vi "Magnet Gap Tester (FPGA).vi"() -> ()   [LabVIEW 2019]
uses:
  <vilib>/Platform/TimedLoop/XDataNode/wakeup.ctl
  <vilib>/Platform/TimedLoop/XDataNode/XDNodeRunTimeDep.lvlib
  <vilib>/Platform/TimedLoop/XDataNode/nitl_modes.ctl
  <vilib>/Platform/TimedLoop/XDataNode/timing_clust.ctl
  <vilib>/Platform/TimedLoop/XDataNode/XDataNode.xnode
  <vilib>/eio/EIONode/EIONode.xnode
  <vilib>/rvi/eio/common/nirviEmuTemplateMethod_errors.vi
  <vilib>/rvi/DataTransferAndStorage/Container/XNode/niFpgaContainer.xnode
  <vilib>/rvi/interface/RandomDataEmulation/nirviRandomDataFpgaReadWriteTemplate.vi
  <vilib>/eio/EIOMethodNode/EIOMethodNode.xnode
  Controls/i2c_state.ctl
panel:
  in  "Samples to Avg":i16=10
  out "AI0":fxp<+/-,24,5>
  in  "Execute":bool
  in  "HalfCycle(Ticks)":u32=200
  in  "i2c_State":T1=enum."W_To_Device"
  in  "Address":u8 format="%08x"
  in  "10-bitAddress":u8 format="%08b"
  in  "TransmitDelay(Ticks)":u32=1000
  in  "Use_10-Bit_Address":bool
  in  "StartStopDelay(Ticks)":u32=1200
  in  "PostAddressDelay(Ticks)":u32=1200
  in  "NumBytesToWrite":i32
  in  "NumBytesToRead":i32
  out "error":errorcluster
  out "Status":i16
  in  "CMD/Param":u8 format="%.0x"
  out "Data":u8 format="%.0x"
  in  "MemoryAddress":u32
  in  "GetRead":bool
  in  "UpdateWrite":bool
  out "REV OUT":bool
  out "FWD OUT":bool
  in  "Reverse":bool
  in  "Forward":bool
  in  "Motor Stop Offset":i32=589
  in  "REV Limit":i32=589
  in  "FWD Limit":i32=589
  out "AI0 (avg)":fxp<+/-,24,5> format="%.4g"
  in  "AI Loop (uSec)":u32
  out "AI Loop Actual":u32=20
  in  "Position Reset":bool
  out "Position (Counts)":i32=589
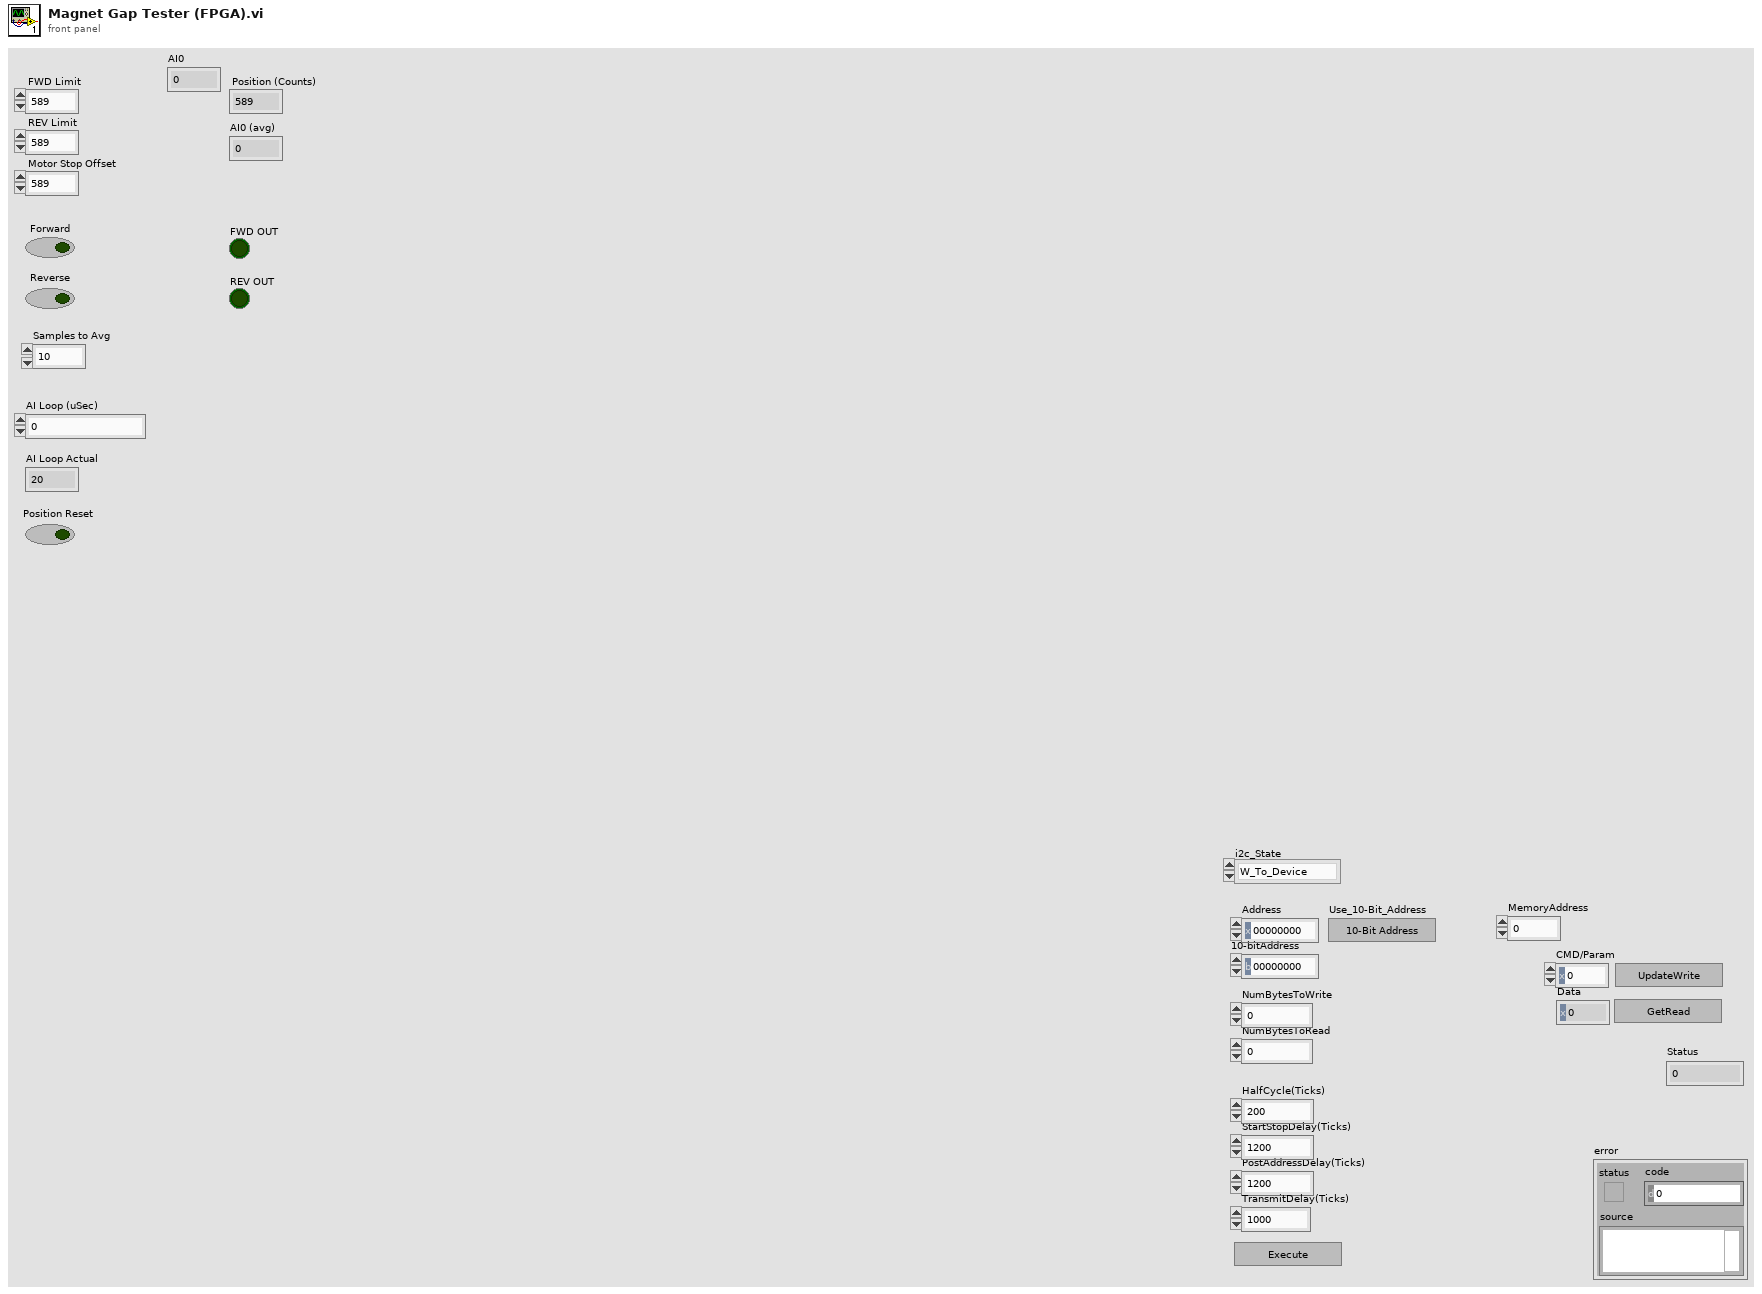
[diagram p1: front panel]
types:
  T1 = typedef "i2c_state.ctl" = enum16{"Monitor", "W_To_Device", "R_From_Device", "W/R_From_Device", "TerminateCore"}
  T2 = typedef "XDNodeRunTimeDep.lvlib/timing_clust.ctl" = cluster{"Expected End [f-1]":u64, "Actual End [f-1]":u64, "Finished Late? [f-1]":bool, "Expected End [i-1]":u64, "Actual End [i-1]":u64, "Finished Late? [i-1]":bool, "Expected Start [i]":u64, "Actual Start [i]":u64, "Expected Start [f]":u64, "Actual Start [f]":u64, "Source Name":string, "Structure Name":string, "Period":i64, "Deadline":i64, "Offset":i64, "Start":i64, "Priority":i32, "Timeout":i32, "Mode":T3, "Wakeup Reason":T4, "Error":errorcluster, "Source Type":string, "Secondary Source Type":string, "Global End Time":u64, "Global Start Time":u64, "Frame Duration":u64, "Iteration Duration":u64, "Assigned CPU":i32, "I/O Scan Engine Mode":u32}
  T3 = typedef "XDNodeRunTimeDep.lvlib/nitl_modes.ctl" = enum32{"No Change", "Process missed periods, maintain original phase", "Discard missed periods, maintain original phase", "Process missed periods, ignore original phase", "Discard missed periods, ignore original phase"}
  T4 = typedef "XDNodeRunTimeDep.lvlib/wakeup.ctl" = enum32{"Normal", "Aborted", "Asynchronous wakeup", "Timing source error", "Timed loop error", "Timeout"}
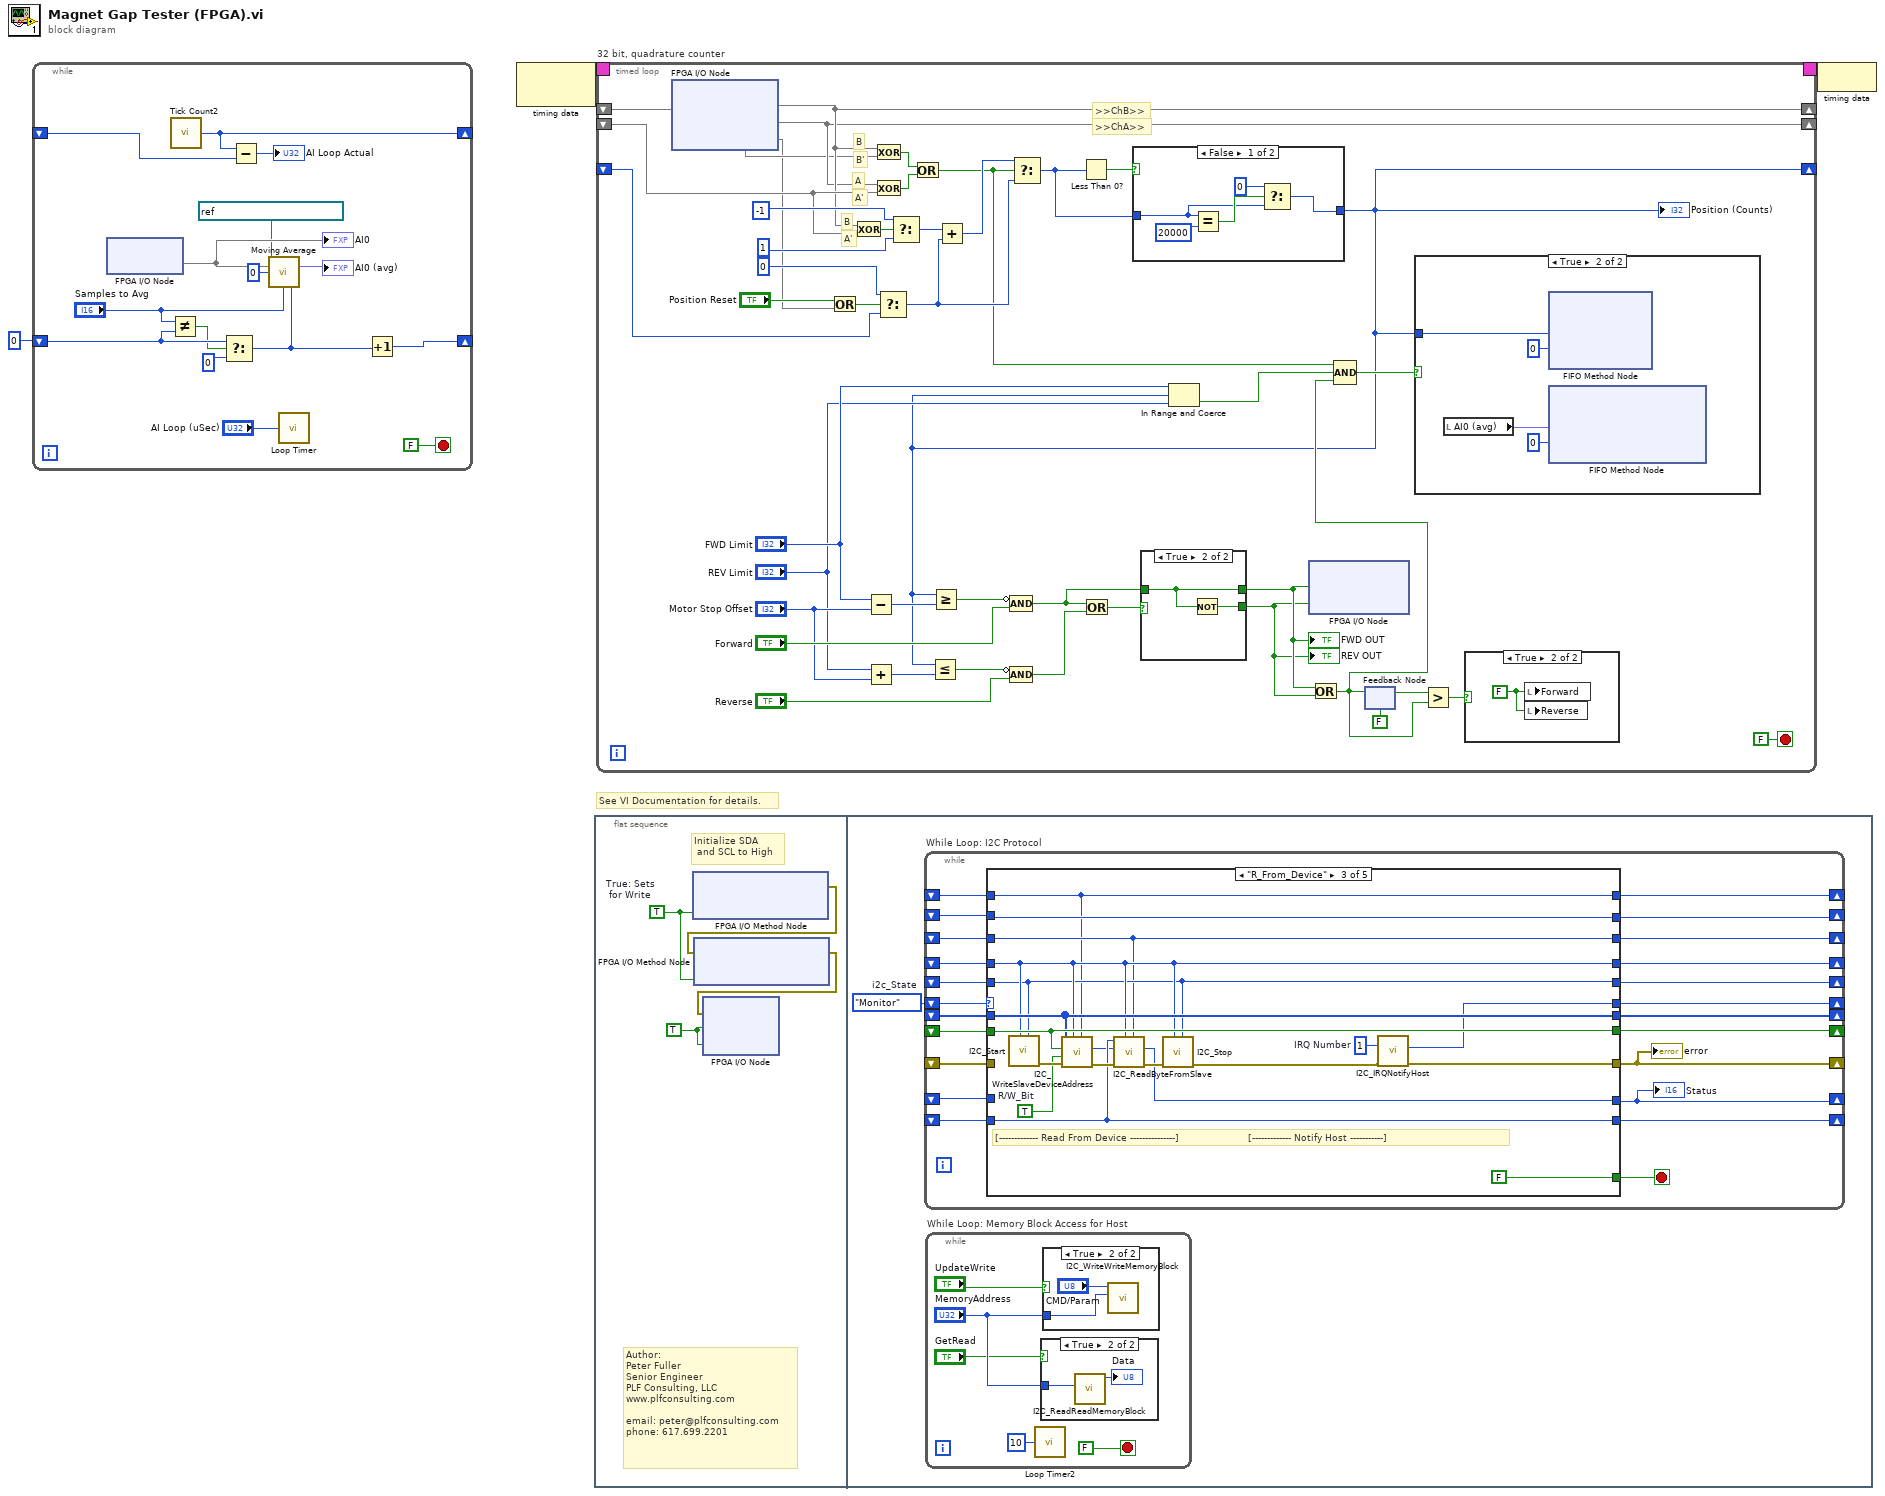
[diagram p0: block diagram]
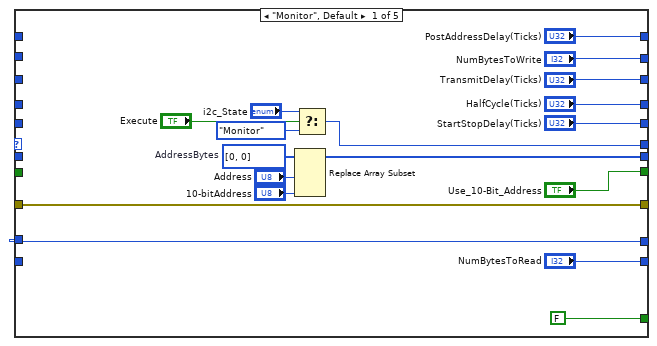
[diagram p4: hidden frame]
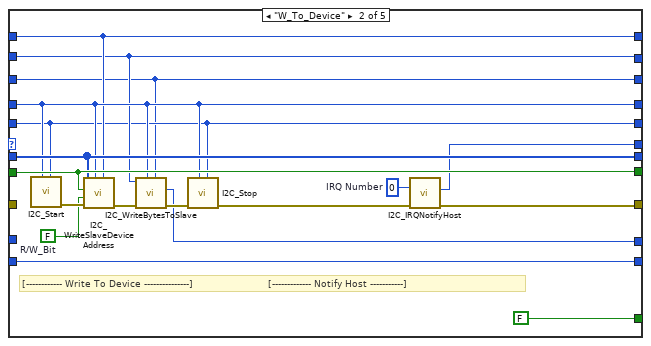
[diagram p5: hidden frame]
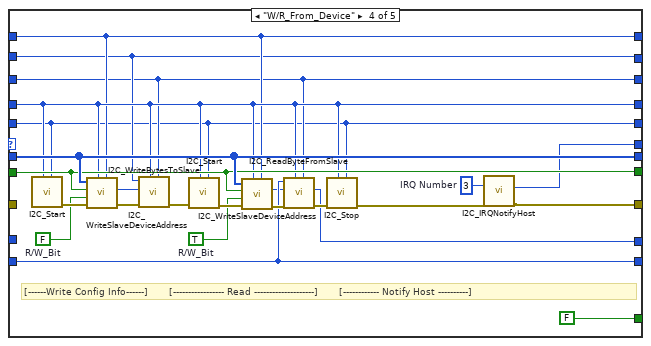
[diagram p6: hidden frame]
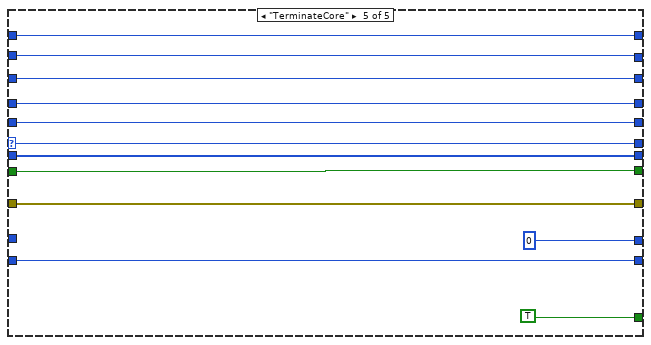
[diagram p7: hidden frame]
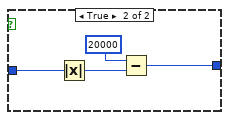
[diagram p11: hidden frame]
diagram:
  # "See VI Documentation for details."
  n1 = while {
    shift-right: [w16] -> _
    shift-left: _ -> [w15]
    shift-right: [w8] -> _
    shift-left: i16 0 ("Moving Point Index") -> [w7]
    stop <- FALSE stop-if-true
    n2 = xnode "FPGA I/O Node"() -> ("AI0"=w13)  [unwired: 1 in, 1 out]
    "AI0" <- w13
    n3 = Not Equal?(x="Samples to Avg", y=w7) -> (x != y?=w5:bool)
    n4 = call "Tick Count2"() -> ("Tick Count(uSec)"=w16:u32)
    n5 = Select(t=w7, s=w5, f=i16 0) -> (s? t:f=w9:i16)
    n6 = Subtract(x=w16, y=w15) -> (x-y=→"AI Loop Actual":u32)
    n7 = call "Moving Average.vi"("Memory In"=refnum<k21> "Running Avg Memory", "N (# of Ave Pts 127 max)"="Samples to Avg", "Moving Point Index"=w9, "Data IN"=w13, "Channel#"=i16 0) -> ("Averaged Data"=→"AI0 (avg)":fxp<+/-,28,17>)  [unwired: 10 in]
    n8 = call "Loop Timer"("Count(uSec)"="AI Loop (uSec)") -> ()  [unwired: 1 out]
    n9 = Increment(x=w9) -> (x+1=w8:i16)
  }
  n10 = node-c288() -> (w3:T2)  [unwired: 1 in]
  n11 = flat-sequence {
    frame #0 {
      w20 = TRUE  # True: Sets   for Write
      w22 = TRUE ("SDA")
      # "Author:\nPeter Fuller\nSenior Engineer\nPLF Consulting, LLC\nwww.plfconsulting.com\n\nemail: peter@plfconsulting.com\nphone: 617.699.2201"
      # "Initialize SDA\n and SCL to High"
      n12 = xnode "FPGA I/O Method Node"("Enable"=w20) -> ("error out"=w21:errorcluster)  [unwired: 2 in, 1 out]
      n13 = xnode "FPGA I/O Method Node"("error in"=w21, "Enable"=w20) -> ("error out"=w19:errorcluster)  [unwired: 1 in, 1 out]
      n14 = xnode "FPGA I/O Node"("error in"=w19, "SDA"=w22, "SCL"=w22) -> ()  [unwired: 2 in, 3 out]
    }
    frame #1 {
      w23 = i2c_state."Monitor"  # i2c_State
      n15 = while "While Loop: I2C Protocol" {
        shift-right: [w50] -> _
        shift-left: w23 -> [w51]
        shift-right: [w54] -> _
        shift-left: _ -> [w55]
        shift-right: [w35] -> _
        shift-left: _ -> [w53]
        shift-right: [w49] -> _
        shift-left: _ -> [w52]
        shift-right: [w48] -> _
        shift-left: _ -> [w47]
        shift-right: [w46] -> _
        shift-left: _ -> [w45]
        shift-right: [w43] -> _
        shift-left: _ -> [w39]
        shift-right: [w42] -> _
        shift-left: _ -> [w38]
        shift-right: [w41] -> _
        shift-left: _ -> [w36]
        shift-right: [w40] -> _
        shift-left: _ -> [w37]
        shift-right: [w34] -> _
        shift-left: _ -> [w33]
        stop <- w44 stop-if-true
        n16 = case shown="\"R_From_Device\"" w51 {
          selector: w51 -> [_ _ _ _ w139]
          tunnel: ["HalfCycle(Ticks)" w88 w105 w126 w141] -> w54
          tunnel: w55 -> [_ w88 w105 w126 w141]
          tunnel: [w69 w83 w92 w111 w139] -> w50
          tunnel: w53 -> [w57 _ _ _ w145]
          tunnel: [w57 w76 w93 w112 w145] -> w35
          tunnel: w52 -> [_ w89 w108 w131 w138]
          tunnel: [w65 w89 w108 w131 w138] -> w49
          tunnel: ["Use_10-Bit_Address" w90 w109 w130 w137] -> w48
          tunnel: w47 -> [_ w90 w109 w130 w137]
          tunnel: ["TransmitDelay(Ticks)" w77 w99 w119 w142] -> w46
          tunnel: w45 -> [_ w77 w99 w119 w142]
          tunnel: [FALSE FALSE FALSE FALSE TRUE] -> w44
          tunnel: w38 -> [_ w80 w102 w121 w143]
          tunnel: w37 -> [_ w79 w101 w120 w136]
          tunnel: w36 -> [_ w78 w100 w118 w140]
          tunnel: ["PostAddressDelay(Ticks)" w81 w98 w122 w144] -> w43
          tunnel: ["NumBytesToWrite" w80 w102 w121 w143] -> w42
          tunnel: ["StartStopDelay(Ticks)" w78 w100 w118 w140] -> w41
          tunnel: ["NumBytesToRead" w79 w101 w120 w136] -> w40
          tunnel: w39 -> [_ w81 w98 w122 w144]
          tunnel: [w56 w75 w97 w117 i16 0 ("Status")] -> w34
          tunnel: w33 -> [w56 _ _ _ _]
          frame "Monitor", Default {
            w68 = u8[] [0, 0]  # AddressBytes
            n17 = Replace Array Subset(array=w68, new element #1="Address", new element #2="10-bitAddress") -> (w65:u8[])  [unwired: 2 in]
            n18 = Select(t="i2c_State", s="Execute", f=i2c_state."Monitor") -> (s? t:f=w69:T1)
          }
          frame "W_To_Device" {
            w74 = u8 0  # IRQ Number
            w84 = FALSE  # R/W_Bit
            # "[------------ Write To Device ---------------]                         [------------- Notify Host -----------]"
            n19 = call "I2C_Start.vi"("TransmitDelay(Ticks)"=w78, "HalfCycle(Ticks)"=w88) -> ("error out"=w87:errorcluster)  [unwired: 2 in, 7 out]
            n20 = call "I2C_WriteSlaveDeviceAddress.vi"("PostAddressDelay(Ticks)"=w81, "HalfCycle(Ticks)"=w88, "error in"=w87, "R/W_Bit"=w84, "10-Bit Address"=w90, "AddressBits"=w89) -> ("error out"=w91:errorcluster)  [unwired: 5 out]
            n21 = call "I2C_WriteBytesToSlave.vi"("InterByteTransmitDelay(Ticks)"=w77, "HalfCycle(Ticks)"=w88, "error in"=w91, "NumBytesToWrite"=w80) -> ("error out"=w86:errorcluster, "Status"=w75:i16)  [unwired: 1 in, 5 out]
            n22 = call "I2C_Stop.vi"("TransmitDelay(Ticks)"=w78, "HalfCycle(Ticks)"=w88, "error in"=w86) -> ("error out"=w82:errorcluster)  [unwired: 1 in, 7 out]
            n23 = call "I2C_IRQNotifyHost.vi"("error out in"=w82, "IRQ Number"=w74) -> ("error out"=w76:errorcluster, "i2c_State"=w83:T1)  [unwired: 8 out]
          }
          frame "R_From_Device" {
            w95 = u8 1  # IRQ Number
            w103 = TRUE  # R/W_Bit
            # "[------------- Read From Device ---------------]                       [------------- Notify Host -----------]"
            n24 = call "I2C_Start.vi"("TransmitDelay(Ticks)"=w100, "HalfCycle(Ticks)"=w105) -> ("error out"=w107:errorcluster)  [unwired: 2 in, 7 out]
            n25 = call "I2C_WriteSlaveDeviceAddress.vi"("PostAddressDelay(Ticks)"=w98, "HalfCycle(Ticks)"=w105, "error in"=w107, "R/W_Bit"=w103, "10-Bit Address"=w109, "AddressBits"=w108) -> ("error out"=w110:errorcluster, "Status"=w96:i16)  [unwired: 4 out]
            n26 = call "I2C_ReadByteFromSlave.vi"("InterByteTransmitDelay(Ticks)"=w99, "HalfCycle(Ticks)"=w105, "error in"=w110, "StatusIn"=w96, "NumBytesToRead"=w101) -> ("error out"=w106:errorcluster, "Status"=w97:i16)  [unwired: 5 out]
            n27 = call "I2C_Stop.vi"("TransmitDelay(Ticks)"=w100, "HalfCycle(Ticks)"=w105, "error in"=w106) -> ("error out"=w94:errorcluster)  [unwired: 1 in, 7 out]
            n28 = call "I2C_IRQNotifyHost.vi"("error out in"=w94, "IRQ Number"=w95) -> ("error out"=w93:errorcluster, "i2c_State"=w92:T1)  [unwired: 8 out]
          }
          frame "W/R_From_Device" {
            w114 = u8 3  # IRQ Number
            w123 = TRUE  # R/W_Bit
            w124 = FALSE  # R/W_Bit
            # "[------Write Config Info------]       [----------------- Read --------------------]       [------------ Notify Host ----------]"
            n29 = call "I2C_Start.vi"("TransmitDelay(Ticks)"=w118, "HalfCycle(Ticks)"=w126) -> ("error out"=w134:errorcluster)  [unwired: 2 in, 7 out]
            n30 = call "I2C_WriteSlaveDeviceAddress.vi"("PostAddressDelay(Ticks)"=w122, "HalfCycle(Ticks)"=w126, "error in"=w134, "R/W_Bit"=w124, "10-Bit Address"=w130, "AddressBits"=w131) -> ("error out"=w127:errorcluster, "Status"=w116:i16)  [unwired: 4 out]
            n31 = call "I2C_WriteBytesToSlave.vi"("InterByteTransmitDelay(Ticks)"=w119, "HalfCycle(Ticks)"=w126, "error in"=w127, "StatusIn"=w116, "NumBytesToWrite"=w121) -> ("error out"=w128:errorcluster)  [unwired: 6 out]
            n32 = call "I2C_Start.vi"("TransmitDelay(Ticks)"=w118, "HalfCycle(Ticks)"=w126, "error in"=w128) -> ("error out"=w132:errorcluster)  [unwired: 1 in, 7 out]
            n33 = call "I2C_WriteSlaveDeviceAddress.vi"("PostAddressDelay(Ticks)"=w122, "HalfCycle(Ticks)"=w126, "error in"=w132, "R/W_Bit"=w123, "10-Bit Address"=w130, "AddressBits"=w131) -> ("error out"=w129:errorcluster, "Status"=w115:i16)  [unwired: 4 out]
            n34 = call "I2C_ReadByteFromSlave.vi"("InterByteTransmitDelay(Ticks)"=w119, "HalfCycle(Ticks)"=w126, "error in"=w129, "StatusIn"=w115, "NumBytesToRead"=w120) -> ("error out"=w133:errorcluster, "Status"=w117:i16)  [unwired: 5 out]
            n35 = call "I2C_Stop.vi"("TransmitDelay(Ticks)"=w118, "HalfCycle(Ticks)"=w126, "error in"=w133) -> ("error out"=w113:errorcluster)  [unwired: 1 in, 7 out]
            n36 = call "I2C_IRQNotifyHost.vi"("error out in"=w113, "IRQ Number"=w114) -> ("error out"=w112:errorcluster, "i2c_State"=w111:T1)  [unwired: 8 out]
          }
          frame "TerminateCore" {
          }
        }
        "error" <- w35
        "Status" <- w34
      }
      n37 = while "While Loop: Memory Block Access for Host" {
        stop <- FALSE stop-if-true
        n38 = call "Loop Timer2"("Count(Ticks)"=u16 10) -> ()  [unwired: 1 out]
        n39 = case shown="True" "GetRead" {
          tunnel: "MemoryAddress" -> [_ w30]
          frame False {
          }
          frame True {
            n40 = call "I2C_ReadReadMemoryBlock.vi"("MemoryAddress"=w30) -> ("Data"=→"Data":u8)  [unwired: 1 in, 9 out]
          }
        }
        n41 = case shown="True" "UpdateWrite" {
          tunnel: "MemoryAddress" -> [_ w32]
          frame False {
          }
          frame True {
            n42 = call "I2C_WriteWriteMemoryBlock.vi"("MemoryAddress"=w32, "Data"="CMD/Param") -> ()  [unwired: 1 in, 9 out]
          }
        }
      }
    }
  }
  n43 = timed-loop "32 bit, quadrature counter" {
    shift-right: [w178] -> _
    shift-left: _ -> [w175]
    shift-right: [w148] -> _
    shift-left: _ -> [w174]
    shift-right: [w177] -> _
    shift-left: _ -> [w179]
    timing: w3 -> [_]
    timing-out: [_] -> w2
    stop <- FALSE ("stop") stop-if-true
    # "A'"
    # "B"
    # "A'"
    # "A"
    # "B'"
    # "B"
    # ">>ChB>>"
    # ">>ChA>>"
    n44 = xnode "FPGA I/O Node"() -> ("RMC/DIO49"=w178, "RMC/DIO48"=w177, "RMC/DIO50"=w170)  [unwired: 3 in, 3 out]
    n45 = Or(x="Position Reset", y=w170) -> (x .or. y?=w169:bool)
    n46 = Exclusive Or(1:w179, 2:w178) -> (0:w180:bool)
    n47 = Subtract(x="FWD Limit", y="Motor Stop Offset") -> (x-y=w168:i32)
    n48 = Add(x="REV Limit", y="Motor Stop Offset") -> (x+y=w165:i32)
    n49 = Exclusive Or(1:w175, 2:w178) -> (0:w181:bool)
    n50 = Exclusive Or(1:w179, 2:w177) -> (0:w182:bool)
    n51 = Select(t=0 ("32 bit"), s=w169, f=w174) -> (s? t:f=w186:i32)
    n52 = Select(t=-1 ("32 bit"), s=w180, f=1 ("32 bit")) -> (s? t:f=w185:i32)
    n53 = Or(x=w181, y=w182) -> (x .or. y?=w155:bool)
    n54 = Add(x=w185, y=w186) -> (x+y=w188:i32)
    n55 = Select(t=w188, s=w155, f=w186) -> (s? t:f=w172:i32)
    n56 = Less Than 0?(x=w172) -> (x < 0?=w173:bool)
    n57 = case shown="False" w173 {
      tunnel: w172 -> [w199 w205]
      tunnel: [w197 w202] -> w148
      frame False {
        n58 = Equal?(x=w199, y=20000) -> (x = y?=w200:bool)
        n59 = Select(t=0, s=w200, f=w199) -> (s? t:f=w197:i32)
      }
      frame True {
        n60 = Absolute Value(x=w205) -> (abs(x)=w204:i32)
        n61 = Subtract(x=20000, y=w204) -> (x-y=w202:i32)
      }
    }
    "Position (Counts)" <- w148
    n62 = Less Or Equal?(x=w148, y=w165) -> (x <= y?=w151:bool)
    n63 = Greater Or Equal?(x=w148, y=w168) -> (x >= y?=w152:bool)
    n64 = Compound Arithmetic op=AND(invert w152, "Forward") -> (w161:bool)
    n65 = Compound Arithmetic op=AND(invert w151, "Reverse") -> (w163:bool)
    n66 = Or(x=w161, y=w163) -> (x .or. y?=w162:bool)
    n67 = case shown="True" w162 {
      tunnel: [w190 w192] -> w160
      tunnel: w161 -> [w190 w192]
      tunnel: [w190 w191] -> w159
      frame False {
      }
      frame True {
        n68 = Not(x=w192) -> (.not. x?=w191:bool)
      }
    }
    "FWD OUT" <- w160
    "REV OUT" <- w159
    n69 = In Range and Coerce(upper limit="FWD Limit", x=w148, lower limit="REV Limit") -> (In Range?=w147:bool)  [unwired: 1 out]
    n70 = xnode "FPGA I/O Node"("RMC/DIO0"=w160, "RMC/DIO1"=w159) -> ()  [unwired: 2 in, 2 out]
    n71 = Or(x=w160, y=w159) -> (x .or. y?=w153:bool)
    n72 = Compound Arithmetic op=AND(w155, w147, w153) -> (w154:bool)
    n73 = feedback-in #1(w153) -> ()
    n74 = feedback #1(FALSE) -> (w157:bool)
    n75 = case shown="True" w154 {
      tunnel: w148 -> [_ w195]
      frame False {
      }
      frame True {
        n76 = local read "AI0 (avg)"() -> (w196:fxp<+/-,24,5>)
        n77 = xnode ("FIFO Method Node")("Element"=w195, "Timeout"=0) -> ()  [unwired: 1 in, 2 out]
        n78 = xnode ("FIFO Method Node")("Element"=w196, "Timeout"=0) -> ()  [unwired: 1 in, 2 out]
      }
    }
    n79 = Greater?(x=w157, y=w153) -> (0:w156:bool)
    n80 = case shown="True" w156 {
      frame False {
      }
      frame True {
        w189 = FALSE
        n81 = local write "Forward"(w189) -> ()
        n82 = local write "Reverse"(w189) -> ()
      }
    }
  }
  n83 = node-c288(w2) -> ()
